vi "wait on settle.vi"(7 "exp exec in":T1={"data file"={"autosave"=FALSE, "File refnum"=refnum, "data file path"=path ""}, "T log file"={"File refnum"=refnum, "T log file path"=path "", "exists"=FALSE}, "exp seq"={"wave params"={"Num of avg"=0, "Num points"=0, "Meas rate (Hz)"=0.0}, "Setpoints"=[], "#"=0, "index"=0, "elapsed time (s)"=0.0, "set time (s)"=0.0, "min settle (s)"=30.0, " Exec Status"=enum."Settling"}, "error"={"status"=FALSE, "code"=0, "source"=""}}) -> (8 "exp exec out":T1={"data file"={"autosave"=FALSE, "File refnum"=refnum, "data file path"=path ""}, "T log file"={"File refnum"=refnum, "T log file path"=path "", "exists"=FALSE}, "exp seq"={"wave params"={"Num of avg"=0, "Num points"=0, "Meas rate (Hz)"=0.0}, "Setpoints"=[], "#"=0, "index"=0, "elapsed time (s)"=0.0, "set time (s)"=0.0, "min settle (s)"=30.0, " Exec Status"=enum."Settling"}, "error"={"status"=FALSE, "code"=0, "source"=""}})   [LabVIEW 2019]
doc: "This subVI waits for the DAQ state machine to report that the temperature is settled before proceeding to the measurement.\n\nPaul K Dixon\nP3600\nCSUSB Physics"
uses:
  typedefs/PID exec cluster.ctl
  typedefs/data file info.ctl
  typedefs/bug temp file info.ctl
  typedefs/exp seq cluster.ctl
  typedefs/wvfm acq params.ctl
  typedefs/bug meas status.ctl
  typedefs/temp mode enum.ctl
  globals/Bug globals.vi
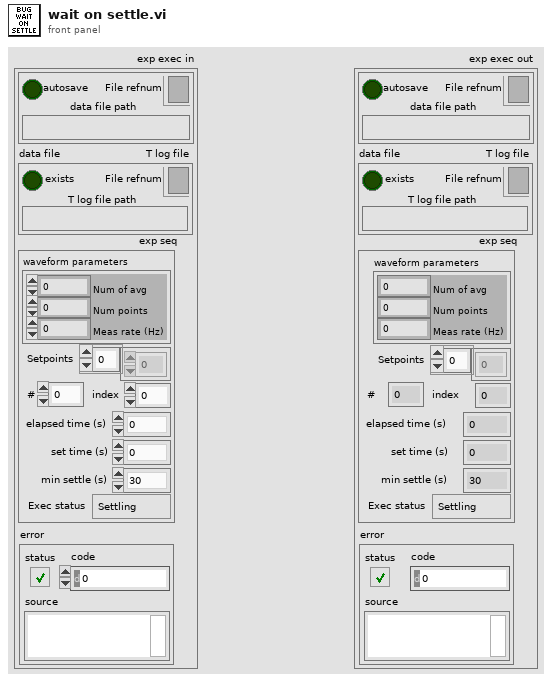
[diagram p1: front panel]
types:
  T1 = typedef "PID exec cluster.ctl" = cluster{"data file":T2, "T log file":T3, "exp seq":T4, "error":errorcluster}
  T2 = typedef "data file info.ctl" = cluster{"autosave":bool, "File refnum":refnum<file>, "data file path":path}
  T3 = typedef "bug temp file info.ctl" = cluster{"File refnum":refnum<file>, "T log file path":path, "exists":bool}
  T4 = typedef "exp seq cluster.ctl" = cluster{"wave params":T5, "Setpoints":dbl[], "#":i32, "index":i32, "elapsed time (s)":dbl, "set time (s)":dbl, "min settle (s)":dbl, " Exec Status":T6}
  T5 = typedef "wvfm acq params.ctl" = cluster{"Num of avg":i32, "Num points":i32, "Meas rate (Hz)":dbl}
  T6 = typedef "bug meas status.ctl" = enum32{"Settling", "Measuring", "Holding", "Exit"}
  T7 = typedef "temp mode enum.ctl" = enum16{"settling", "measuring", "holding", "Exit"}
  T8 = typedef "temp cont cluster.ctl" = cluster{"T exec":T9, "T status":T10, "T params":T12, "utility":T13}
  T9 = typedef "temp exec cluster.ctl" = cluster{"T mode":T7, "exec setpoint":dbl, "reset":bool, "man power":dbl, "man":bool, "log":bool, "clear":bool}
  T10 = typedef "temp indicator.ctl" = cluster{"Control status":T11, "Temp":dbl, "Power":dbl, "Time in settle band":dbl, "Settled":bool, "Low":bool, "High":bool, "Setpoint":dbl, "Control":bool, "In Settle Band":bool}
  T11 = typedef "temp control status.ctl" = enum16{"In Settle Band", "In Control Band", "Below Control Band", "Above Control Band"}
  T12 = typedef "PID control parameters.ctl" = cluster{"Setpoint":dbl, "Control Bandwidth":dbl, "Integral Time":dbl, "Int\nON":bool, "Derivative Tme":dbl, "Der\nON":bool, "Settle Bandwidth":dbl, "Settle Time":dbl}
  T13 = typedef "temp cont utility.ctl" = cluster{"meas index":i32, "wait (ms)":i32, "H Vmax":dbl, "power out":dbl, "heat volt out":dbl, "heat volt in":dbl, "therm volt":dbl, "t T P hist":dbl[][], "cont hist":dbl[][]}
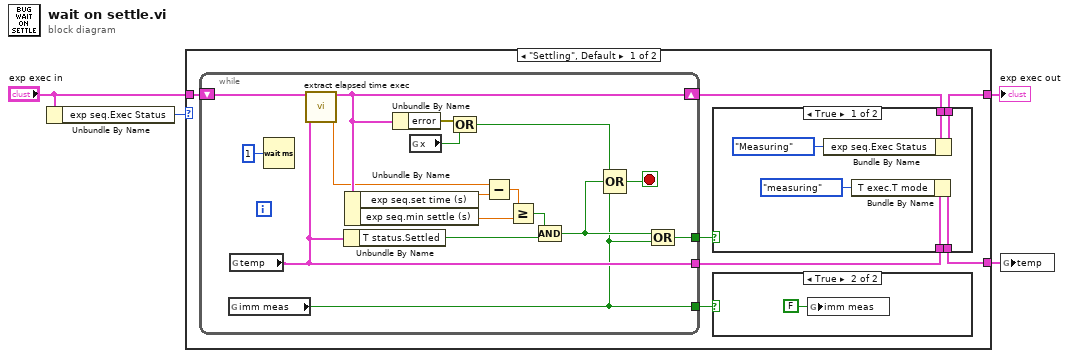
[diagram p0: block diagram]
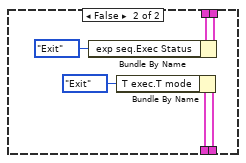
[diagram p3: hidden frame]
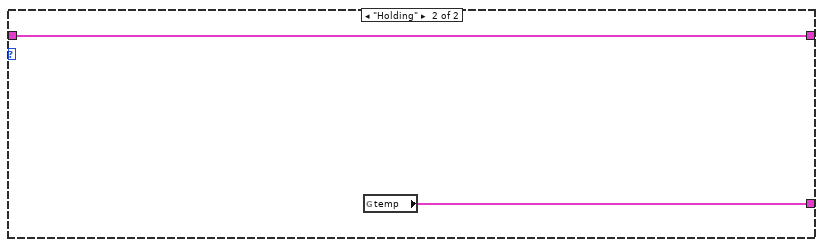
[diagram p4: hidden frame]
diagram:
  n1 = Unbundle By Name("exp exec in") -> ("exp seq.Exec Status"=w1:T6)
  n2 = case shown="\"Settling\", Default" w1 {
    tunnel: [w9 w43] -> w4
    tunnel: [w7 w42] -> w3
    tunnel: "exp exec in" -> [w11 w43]
    frame "Settling", Default {
      n3 = while {
        shift-right: [w38] -> w10
        shift-left: w11 -> [w39]
        tunnel: [w25] -> w6
        tunnel: [w29] -> w8
        tunnel: [w26] -> w5
        stop <- w28 stop-if-true
        n4 = global read "Bug globals.vi" "imm meas"() -> (w26:bool)
        n5 = global read "Bug globals.vi" "temp"() -> (w29:T8)
        n6 = Wait (ms)(milliseconds to wait=u32 1) -> ()  [unwired: 1 out]
        n7 = call "extract elapsed time exec.vi"("exp exec"=w39, "temp"=w29) -> ("exec out"=w38:T1, "latest time (s)"=w36:dbl)  [unwired: 12 in]
        n8 = Unbundle By Name(w29) -> ("T status.Settled"=w33:bool)
        n9 = Unbundle By Name(w38) -> ("exp seq.set time (s)"=w37:dbl, "exp seq.min settle (s)"=w35:dbl)
        n10 = Unbundle By Name(w38) -> ("error"=w41:errorcluster)
        n11 = global read "Bug globals.vi" "x"() -> (w40:bool)
        n12 = Compound Arithmetic op=OR(w41, w40) -> (w31:bool)
        n13 = Subtract(x=w36, y=w37) -> (x-y=w34:dbl)
        n14 = Greater Or Equal?(x=w34, y=w35) -> (x >= y?=w32:bool)
        n15 = Compound Arithmetic op=AND(w32, w33) -> (w27:bool)
        n16 = Compound Arithmetic op=OR(w31, w27, w26) -> (w28:bool)
        n17 = Compound Arithmetic op=OR(w27, w26) -> (w25:bool)
      }
      n18 = case shown="True" w6 {
        tunnel: w10 -> [w18 w24]
        tunnel: [w17 w23] -> w9
        tunnel: w8 -> [w15 w21]
        tunnel: [w14 w20] -> w7
        frame True {
          n19 = Bundle By Name(cluster=w18, "exp seq.Exec Status"=bug_meas_status."Measuring" ("exp seq. Exec Status")) -> (w17:T1)
          n20 = Bundle By Name(cluster=w15, "T exec.T mode"=temp_mode_enum."measuring") -> (w14:T8)
        }
        frame False {
          n21 = Bundle By Name(cluster=w24, "exp seq.Exec Status"=bug_meas_status."Exit" ("exp seq. Exec Status")) -> (w23:T1)
          n22 = Bundle By Name(cluster=w21, "T exec.T mode"=temp_mode_enum."Exit") -> (w20:T8)
        }
      }
      n23 = case shown="True" w5 {
        frame False {
        }
        frame True {
          n24 = global write "Bug globals.vi" "imm meas"(FALSE ("imm meas")) -> ()
        }
      }
    }
    frame "Holding" {
      n25 = global read "Bug globals.vi" "temp"() -> (w42:T8)
    }
  }
  "exp exec out" <- w4
  n26 = global write "Bug globals.vi" "temp"(w3) -> ()
